vi "opencomm.vi"(0 "VISA resource name":refnum<visa-resource-name>="ASRL2::INSTR", 1 "Baud-rate (57600)":u32=57600) -> (2 "duplicate VISA resource name":refnum<visa-resource-name>, 3 "Error":bool)   [LabVIEW 2020]
uses:
  <vilib>/Instr/_visa.llb/VISA Configure Serial Port (Instr).vi
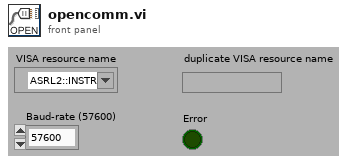
[diagram p1: front panel]
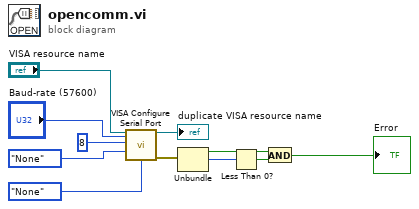
[diagram p0: block diagram]
diagram:
  n1 = call-poly "VISA Configure Serial Port"("VISA resource name"="VISA resource name", "baud rate (9600)"="Baud-rate (57600)", "data bits (8)"=u16 8, "parity (0:none)"=enum16{"None", "Odd", "Even", "Mark", "Space"}."None", "flow control (0:none)"=enum16{"None", "XON/XOFF", "RTS/CTS"}."None" ("flow control (0:None)")) -> ("VISA resource name out"=→"duplicate VISA resource name":refnum<visa-resource-name>, "error out"=w5:errorcluster)  [unwired: 9 in]
  n2 = Unbundle(w5) -> ("status"=w2:bool, "code"=w4:i32)  [unwired: 1 out]
  n3 = Less Than 0?(x=w4) -> (x < 0?=w3:bool)
  n4 = And(x=w2, y=w3) -> (x .and. y?=→"Error":bool)
